vi "Main Editor UI.vi"() -> ()   [LabVIEW 2015, in "E2E Tag Exchange editor node.lvclass"]
doc: "This is the main view for configuration the behavior of a module in the DCAF standard editor."
uses:
  E2E Tag Exchange editor node.lvclass
  <vilib>/NI/Configuration Framework/Node/NodeRef.ctl
  <vilib>/NI/Configuration Framework/Node/NISE_CEF_Node.lvclass
  <vilib>/NI/AMC/Message Queue.ctl
  <vilib>/NI/AMC/Message.ctl
  <vilib>/NI/Tools/Keyed Array/KeyedArray.ctl
  <vilib>/NI/Configuration Framework/Node/StopEvent.ctl
  <vilib>/NI/Configuration Framework/Node/RefreshUIEvent.ctl
  <vilib>/NI/Configuration Framework/Node/CacheState.ctl
  <vilib>/NI/Configuration Framework/Node/NodeChangeEvent.ctl
  <vilib>/NI/DCAF UI Toolkit/Controls/Move One Right.ctl
  <vilib>/NI/DCAF UI Toolkit/Controls/Move All Right.ctl
  <vilib>/NI/DCAF UI Toolkit/Controls/Move One Left.ctl
  <vilib>/NI/DCAF UI Toolkit/Controls/Move All Left.ctl
  module/configuration/Runtime Implementation.ctl
  references.ctl
  Pairing Tab References.ctl
  Tag Exchange Tab References.ctl
  <vilib>/Utility/miscctls.llb/LVPositionTypeDef.ctl
  <vilib>/NI/Tools/Keyed Array/Tools_KeyedArray.lvlib
  <vilib>/NI/AMC/AMC.lvlib
  <vilib>/NI/DCAF UI Toolkit/Controls/DCAF UI Elements.lvlib
  <vilib>/NI/DCAF/Tag Editor Core/Configuration Editor/Classes/Engine Parent/Engine Parent Editor Node.lvclass
  module/configuration/E2E Tag Exchange configuration.lvclass
panel:
  in  "node change":T1
  in  "cache state":T2
  in  "refresh UI":T3
  in  "stop event":T4
  in  "Tab Control":T5(tab)
  in  "Paired Module UID":string
  in  "Unpair":bool
  in  "Pair":bool
  in  "implementation":T6 caption="Runtime Implementation"
  in  "E2E Nodes":i32(listbox)
  in  "From External Engine":i32(listbox)
  in  "To External Engine":i32(listbox)
  in  "Prefix?":bool
  in  "Tag Prefix":string
  in  "Move All Left":T7
  in  "Move One Left":T8
  in  "Move All Right":T9
  in  "Move One Right":T10
  in  "Filter":string
  in  "Available Tag List":i32(listbox)
  in  "main queue":T11
  in  "node ref":T12
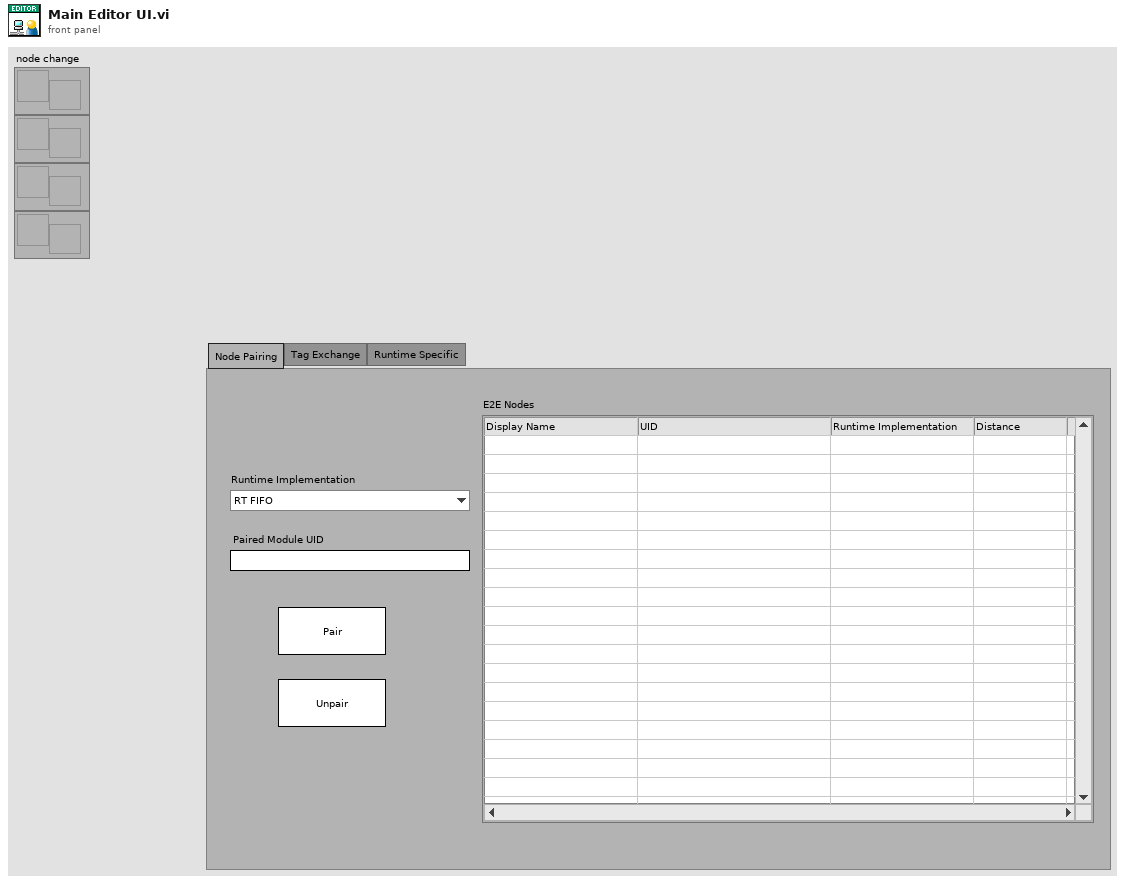
[diagram p1: front panel]
types:
  T1 = typedef "NISE_CEF_Node.lvclass/NodeChangeEvent.ctl" = refnum<user-event>
  T2 = typedef "NISE_CEF_Node.lvclass/CacheState.ctl" = refnum<user-event>
  T3 = typedef "NISE_CEF_Node.lvclass/RefreshUIEvent.ctl" = refnum<user-event>
  T4 = typedef "NISE_CEF_Node.lvclass/StopEvent.ctl" = refnum<user-event>
  T5 = enum32{"Node Pairing", "Tag Exchange", "Runtime Specific"}
  T6 = typedef "E2E Tag Exchange configuration.lvclass/Runtime Implementation.ctl" = enum16{"RT FIFO", "UDP"}
  T7 = typedef "DCAF UI Elements.lvlib/Move All Left.ctl" = bool
  T8 = typedef "DCAF UI Elements.lvlib/Move One Left.ctl" = bool
  T9 = typedef "DCAF UI Elements.lvlib/Move All Right.ctl" = bool
  T10 = typedef "DCAF UI Elements.lvlib/Move One Right.ctl" = bool
  T11 = typedef "AMC.lvlib/Message Queue.ctl" = refnum<queue>
  T12 = typedef "NISE_CEF_Node.lvclass/NodeRef.ctl" = refnum<data-value>
  T13 = typedef "E2E Tag Exchange editor node.lvclass/Tag Exchange Tab References.ctl" = cluster{"Available Tag List":refnum<vi>, "To External Engine":refnum<vi>, "From External Engine":refnum<vi>, "Move One Right":refnum<vi>, "Move All Right":refnum<vi>, "Move One Left":refnum<vi>, "Move All Left":refnum<vi>}
  T14 = typedef "E2E Tag Exchange editor node.lvclass/Pairing Tab References.ctl" = cluster{"E2E Nodes":refnum<vi>, "Pair":refnum<vi>, "Unpair":refnum<vi>, "implementation":refnum<vi>, "Paired Module UID":refnum<vi>}
  T15 = typedef "E2E Tag Exchange editor node.lvclass/references.ctl" = cluster{"stop event":T4, "refresh UI":T3, "cache state":T2, "node change":T1, "main queue":T11}
  T16 = typedef "LVPositionTypeDef.ctl" = cluster{"Left":i32, "Top":i32}
  T17 = typedef "E2E Tag Exchange editor node.lvclass/object references.ctl" = cluster{"engine":refnum<data-value>, "Node Ref":refnum<data-value>}
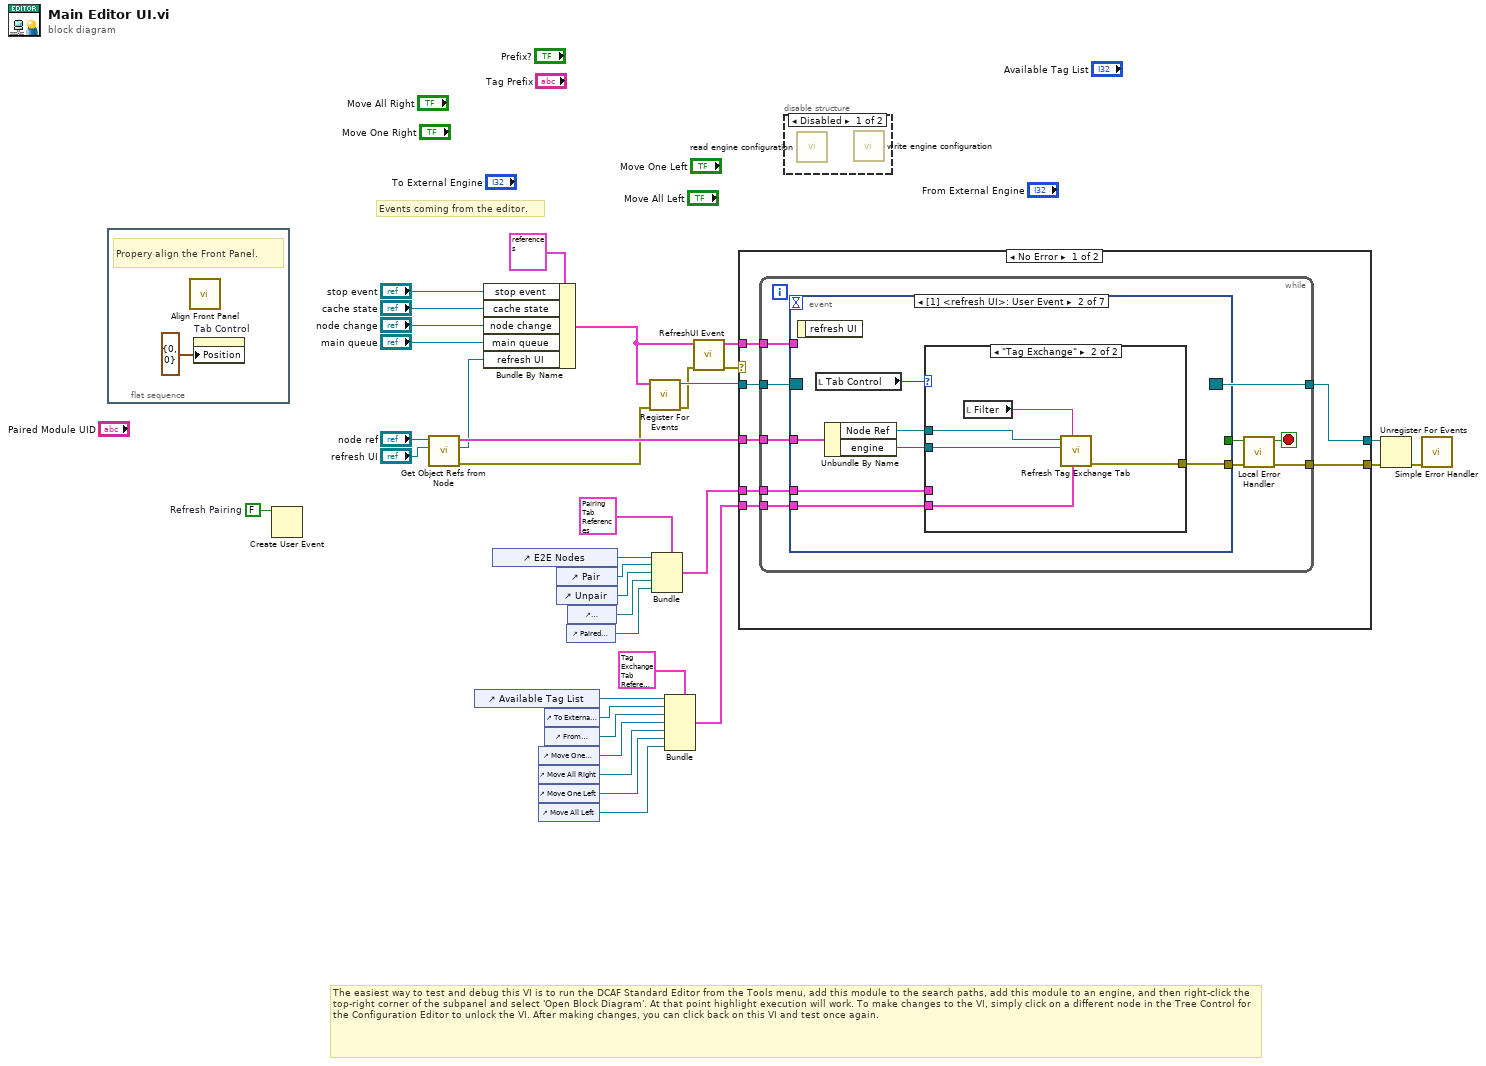
[diagram p0: block diagram]
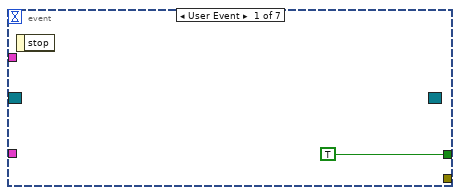
[diagram p3: hidden frame]
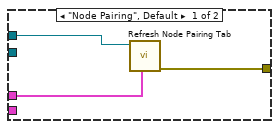
[diagram p4: hidden frame]
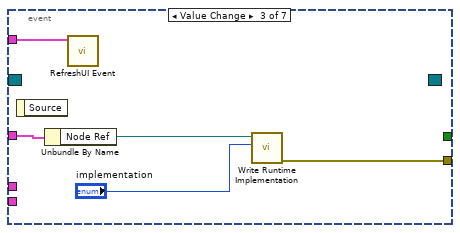
[diagram p5: hidden frame]
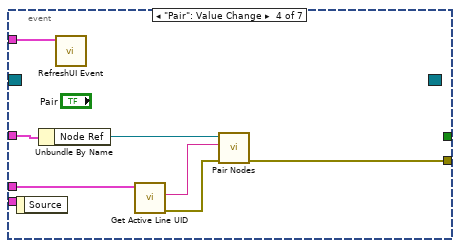
[diagram p6: hidden frame]
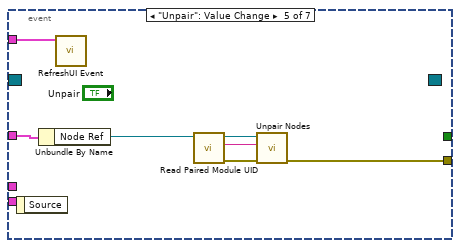
[diagram p7: hidden frame]
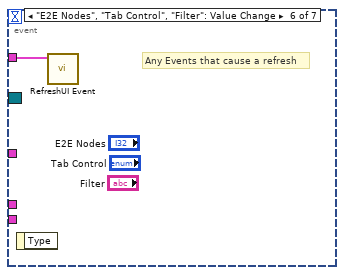
[diagram p8: hidden frame]
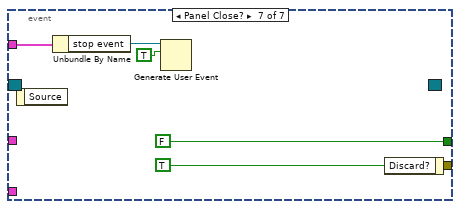
[diagram p9: hidden frame]
diagram:
  w12 = FALSE  # Refresh Pairing
  # "The easiest way to test and debug this VI is to run the DCAF Standard Editor from the Tools menu, add this module to the search paths, add this module to an engine, and then right-click the top-right corner of the subpanel and select 'Open Block Diagram'. At that point highlight execution will work. To make changes to the VI, simply click on a different node in the Tree Control for the Configuration Editor to unlock the VI. After making changes, you can click back on this VI and test once again."
  # "Events coming from the editor."
  n1 = flat-sequence {
    frame #0 {
      # "Propery align the Front Panel."
      n2 = call <vilib>:"Align Front Panel.vi"() -> ()  [unwired: 10 in, 2 out]
      n3 = property on="Tab Control" class="TabCtl (strict)"("Position"=T16 {"Left"=0, "Top"=0}) -> ()  [unwired: 2 in, 2 out]
    }
  }
  n4 = Create User Event(user event datatype=w12) -> ()  [unwired: 1 in, 2 out]
  n5 = call "Get Object Refs from Node.vi"("Refresh UI"="refresh UI", "Data Value Reference in"="node ref") -> ("error out"=w18:errorcluster, "Refresh UI out"=w19:T3, "References"=w23:T17)  [unwired: 7 in]
  n6 = control-ref of="Available Tag List"() -> (w9:refnum<vi>)
  n7 = Bundle By Name(cluster=T15 {"stop event"=refnum, "refresh UI"=refnum, "cache state"=refnum, "node change"=refnum, "main queue"=refnum} ("References"), "stop event"="stop event", "cache state"="cache state", "node change"="node change", "main queue"="main queue", "refresh UI"=w19) -> (w24:T15)
  n8 = control-ref of="E2E Nodes"() -> (w17:refnum<vi>)
  n9 = control-ref of="Move One Right"() -> (w8:refnum<vi>)
  n10 = control-ref of="Move All Right"() -> (w7:refnum<vi>)
  n11 = control-ref of="Move One Left"() -> (w6:refnum<vi>)
  n12 = control-ref of="Move All Left"() -> (w5:refnum<vi>)
  n13 = control-ref of="To External Engine"() -> (w4:refnum<vi>)
  n14 = control-ref of="From External Engine"() -> (w3:refnum<vi>)
  n15 = control-ref of="Pair"() -> (w16:refnum<vi>)
  n16 = control-ref of="Unpair"() -> (w15:refnum<vi>)
  n17 = control-ref of="Paired Module UID"() -> (w10:refnum<vi>)
  n18 = control-ref of="implementation"() -> (w14:refnum<vi>)
  n19 = call "Register For Events.vi"("error in"=w18, "References"=w24) -> ("error out"=w22:errorcluster, "Event Registration Refnum"=w26:refnum<event-registration>)  [unwired: 8 in]
  n20 = Bundle(cluster=T14 {"E2E Nodes"=refnum, "Pair"=refnum, "Unpair"=refnum, "implementation"=refnum, "Paired Module UID"=refnum} ("Pairing Tab References"), "E2E Nodes"=w17, "Pair"=w16, "Unpair"=w15, "implementation"=w14, "Paired Module UID"=w10) -> (w11:T14)
  n21 = Bundle(cluster=T13 {"Available Tag List"=refnum, "To External Engine"=refnum, "From External Engine"=refnum, "Move One Right"=refnum, "Move All Right"=refnum, "Move One Left"=refnum, "Move All Left"=refnum} ("Tag Exchange Tab References"), "Available Tag List"=w9, "To External Engine"=w4, "From External Engine"=w3, "Move One Right"=w8, "Move All Right"=w7, "Move One Left"=w6, "Move All Left"=w5) -> (w1:T13)
  n22 = call "RefreshUI Event.vi"("error in (no error)"=w22, "References in"=w24) -> ("error out"=w21:errorcluster, "References out"=w25:T15)  [unwired: 8 in]
  n23 = case shown="No Error" w21 {
    selector: w21 -> [_ w96]
    tunnel: w26 -> [w43 w95]
    tunnel: [w42 w95] -> w35
    tunnel: [w39 w96] -> w34
    tunnel: w25 -> [w41 _]
    tunnel: w23 -> [w40 _]
    tunnel: w11 -> [w38 _]
    tunnel: w1 -> [w37 _]
    frame No Error {
      n24 = while {
        tunnel: w43 -> [w53]
        tunnel: [w52] -> w42
        tunnel: [w49] -> w39
        tunnel: w41 -> [w47]
        tunnel: w40 -> [w46]
        tunnel: w38 -> [w45]
        tunnel: w37 -> [w44]
        stop <- w51 stop-if-true
        n25 = event shown="[1] <refresh UI>: User Event" {
          selector: w53 -> [_ _ _ _ _ _ _]
          dyn-events: [_ _ _ _ _ _ _] -> w52
          timeout: _ -> [_ _ _ _ _ _ _]
          tunnel: [TRUE _ _ _ _ _ FALSE] -> w50
          tunnel: [_ w61 w74 w79 w86 _ _] -> w48
          tunnel: w47 -> [_ _ w70 w80 w87 w89 w91]
          tunnel: w46 -> [_ w60 w73 w81 w88 _ _]
          tunnel: w45 -> [_ w58 _ w76 _ _ _]
          tunnel: w44 -> [_ w55 _ _ _ _ _]
          event User Event {
            n26 = event-data() -> ()  [unwired: 1 in, 1 out]
          }
          event User Event {
            n27 = event-data() -> ()  [unwired: 1 in, 1 out]
            n28 = local read "Tab Control"() -> (w57:T5)
            n29 = Unbundle By Name(w60) -> ("Node Ref"=w59:refnum<data-value>, "engine"=w56:refnum<data-value>)
            n30 = case shown="\"Tag Exchange\"" w57 {
              tunnel: [w64 w67] -> w61
              tunnel: w59 -> [w62 w69]
              tunnel: w58 -> [w63 _]
              tunnel: w56 -> [_ w68]
              tunnel: w55 -> [_ w65]
              frame "Node Pairing", Default {
                n31 = call "Refresh Node Pairing Tab.vi"("Pairing Tab References"=w63, "E2E editor node in"=w62) -> ("error out"=w64:errorcluster)  [unwired: 8 in, 1 out]
              }
              frame "Tag Exchange" {
                n32 = local read "Filter"() -> (w66:string)
                n33 = call "Refresh Tag Exchange Tab.vi"("Tag Exchange Tab References"=w65, "Filter"=w66, "engine"=w68, "E2E editor node in"=w69) -> ("error out"=w67:errorcluster)  [unwired: 5 in, 2 out]
              }
            }
          }
          event Value Change {
            n34 = event-data() -> ()  [unwired: 1 in, 1 out]
            n35 = Unbundle By Name(w73) -> ("Node Ref"=w72:refnum<data-value>)
            n36 = call "RefreshUI Event.vi"("References in"=w70) -> ()  [unwired: 9 in, 2 out]
            n37 = call "Write Runtime Implementation.vi"("Runtime Implementation"="implementation", "E2E editor node in"=w72) -> ("error out"=w74:errorcluster)  [unwired: 8 in, 1 out]
          }
          event "Pair": Value Change {
            n38 = event-data() -> ()  [unwired: 1 in, 1 out]
            n39 = Unbundle By Name(w81) -> ("Node Ref"=w78:refnum<data-value>)
            n40 = call "RefreshUI Event.vi"("References in"=w80) -> ()  [unwired: 9 in, 2 out]
            n41 = call "Get Active Line UID.vi"("Pairing Tab Refs"=w76) -> ("error out"=w77:errorcluster, "Line UID"=w75:string)  [unwired: 9 in]
            n42 = call "Pair Nodes.vi"("error in (no error)"=w77, "Node UID to Pair"=w75, "E2E editor node in"=w78) -> ("error out"=w79:errorcluster)  [unwired: 7 in, 1 out]
          }
          event "Unpair": Value Change {
            n43 = event-data() -> ()  [unwired: 1 in, 1 out]
            n44 = Unbundle By Name(w88) -> ("Node Ref"=w85:refnum<data-value>)
            n45 = call "RefreshUI Event.vi"("References in"=w87) -> ()  [unwired: 9 in, 2 out]
            n46 = call "Read Paired Module UID.vi"("E2E editor node in"=w85) -> ("error out"=w82:errorcluster, "Paired Module UID"=w83:string, "E2E editor node out"=w84:refnum<data-value>)  [unwired: 8 in]
            n47 = call "Unpair Nodes.vi"("error in (no error)"=w82, "Node UID to Unpair"=w83, "E2E editor node in"=w84) -> ("error out"=w86:errorcluster)  [unwired: 7 in, 1 out]
          }
          event "E2E Nodes", "Tab Control", "Filter": Value Change {
            # "Any Events that cause a refresh"
            n48 = event-data() -> ()  [unwired: 1 in, 1 out]
            n49 = call "RefreshUI Event.vi"("References in"=w89) -> ()  [unwired: 9 in, 2 out]
          }
          event Panel Close? {
            n50 = event-data() -> ()  [unwired: 1 in, 1 out]
            n51 = Unbundle By Name(w91) -> ("stop event"=w90:T4)
            n52 = Generate User Event(user event=w90, event data cluster=TRUE ("event data")) -> ()  [unwired: 2 in, 2 out]
            n53 = event-data("Discard?"=TRUE) -> ()  [unwired: 1 in, 1 out]
          }
        }
        n54 = call "Local Error Handler.vi"("error in"=w48, "Stop in"=w50) -> ("error out"=w49:errorcluster, "Stop out"=w51:bool)  [unwired: 8 in]
      }
    }
    frame Error {
    }
  }
  n55 = disable-structure shown="Disabled" {
    frame Disabled {
      n56 = call <vilib>:"read engine configuration.vi"() -> ()  [unwired: 9 in, 3 out]
      n57 = call <vilib>:"write engine configuration.vi"() -> ()  [unwired: 10 in, 2 out]
    }
    frame Enabled {
    }
  }
  n58 = Unregister For Events(event registration refnum=w35, error in=w34) -> (error out=w33:errorcluster)
  n59 = call <vilib>:"Simple Error Handler.vi"("error in (no error)"=w33) -> ()  [unwired: 4 in, 5 out]
